vi "QR_top_left.vi"(8 "errin":errorcluster, 11 "image":string) -> (0 "error out":errorcluster caption="errout", 3 "Réponse":string, 5 "version":string, 6 "SN":string, 7 "PN":string)   [LabVIEW 2020]
uses:
  <userlib>/Alex.vi/FGV.ctl
  <vilib>/regexp/Match Regular Expression.xnode
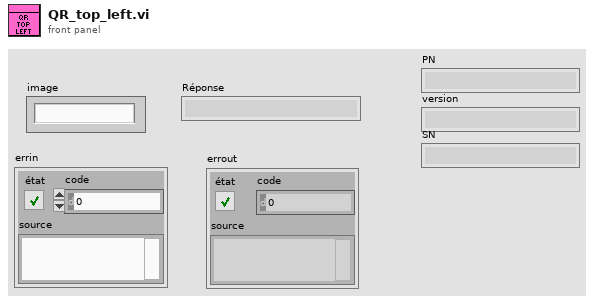
[diagram p1: front panel]
types:
  T1 = typedef "FGV.ctl" = enum16{"GET", "SET", "RAZ"}
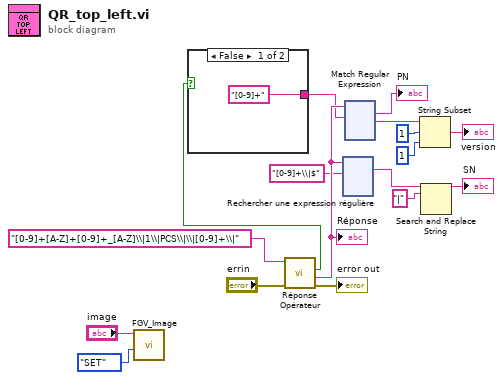
[diagram p0: block diagram]
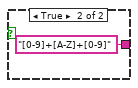
[diagram p2: hidden frame]
diagram:
  n1 = call <userlib>:"FGV_Image.vi"("Énum"=FGV."SET", "IN"="image") -> ()  [unwired: 9 in, 1 out]
  n2 = call "Réponse Opérateur.vi"("errin"="errin", "expression régulière"="[0-9]+[A-Z]+[0-9]+_[A-Z]\\|1\\|PCS\\|\\|[0-9]+\\|") -> ("errout"=→"error out":errorcluster, "toute l'expression"=w7:string, "Standard?"=w1:bool)  [unwired: 6 in, 1 out]
  "Réponse" <- w7
  n3 = case shown="False" w1 {
    tunnel: ["[0-9]+" ("chaîne en entrée") "[0-9]+[A-Z]+[0-9]" ("chaîne en entrée")] -> w2
    frame False {
    }
    frame True {
    }
  }
  n4 = xnode "Rechercher une expression régulière"("chaîne en entrée"=w7, "expression régulière"="[0-9]+\\|$" ("chaîne en entrée")) -> ("toute l'expression"=w5:string)  [unwired: 4 in, 4 out]
  n5 = xnode "Match Regular Expression"("chaîne en entrée"=w7, "expression régulière"=w2) -> ("toute l'expression"=→"PN":string, "après la correspondance"=w11:string)  [unwired: 4 in, 3 out]
  n6 = String Subset(string=w11, offset (0)=1, length (rest)=1 ("longueur (reste)")) -> (substring=→"version":string)
  n7 = Search and Replace String(input string=w5, search string="|" ("chaîne recherchée")) -> (result string=→"SN":string)  [unwired: 6 in, 3 out]
